vi "XYZStage-Request motor Z command.vi"(8 "error in (no error)":errorcluster, 9 "Wait for acknowledge?":bool=TRUE, 10 "Motor Z":sgl) -> (0 "error out":errorcluster, 1 "Timed out while waiting for acknowledgement":bool, 2 "Acknowledgement message":string)   [LabVIEW 2017]
doc: "Sends a request to the XYZ Stage driver to move the motor to the specified position on the Z axis."
uses:
  Typedefs/XYZ stage states.ctl
  Typedefs/XYZ stage data.ctl
  Typedefs/XYZ channel ring.ctl
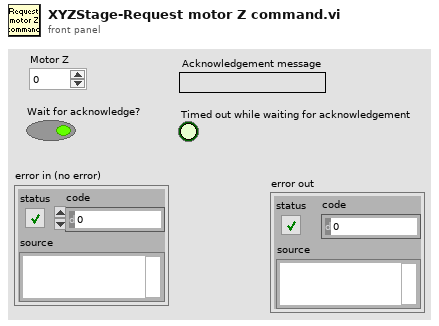
[diagram p1: front panel]
types:
  T1 = typedef "XYZ channel ring.ctl" = string
  T2 = typedef "XYZ stage data.ctl" = cluster{"Command":T3, "Channel":T1, "X":sgl, "Y":sgl, "Z":sgl, "Speed":i32, "Zero":bool, "Use acknowledgement?":bool}
  T3 = typedef "XYZ stage states.ctl" = enum16{"Dequeue", "Initialize", "Read Position", "Read Speed Setting", "Move", "Set Max Speed", "Reset Axis", "Stop all movement"}
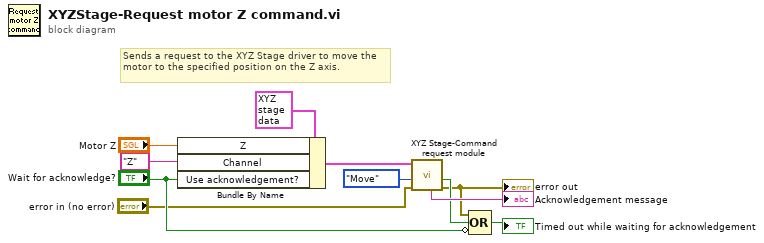
[diagram p0: block diagram]
diagram:
  # "Sends a request to the XYZ Stage driver to move the motor to the specified position on the Z axis."
  n1 = Bundle By Name(cluster=T2 {"Command"=enum."Initialize", "Channel"="", "X"=0.0, "Y"=0.0, "Z"=0.0, "Speed"=0, "Zero"=TRUE, "Use acknowledgement?"=FALSE} ("XYZ Stage data to queue"), "Z"="Motor Z", "Channel"=T1 "Z", "Use acknowledgement?"="Wait for acknowledge?") -> (w11:T2)
  n2 = call "XYZ Stage-Command request module.vi"("error in"="error in (no error)", "Command"=XYZ_stage_states."Move", "XYZ Stage data to queue"=w11) -> ("error out"=w1:errorcluster, "Timed out while waiting for acknowledgement"=w4:bool, "Acknowledgement message"=→"Acknowledgement message":string)  [unwired: 4 in, 2 out]
  "error out" <- w1
  n3 = Compound Arithmetic op=OR(w1, w4, invert "Wait for acknowledge?") -> (→"Timed out while waiting for acknowledgement":bool)
